vi "Configure_SL.vi"() -> (1 "changed?":bool, 2 "Property":string[](array[string]))   [LabVIEW 2019]
uses:
  <vilib>/Utility/miscctls.llb/LVRowAndColumnUnsignedTypeDef.ctl
panel:
  out "Table Control":string[][](table)
  out "error out":errorcluster
  in  "Properties":i32(listbox)=-1
  in  "Cancel":bool
  in  "OK":bool
  # "SystemLink Panel\n\nhttps://www.systemlinkcloud.com\n\nAPI: https://api.systemlinkcloud.com"
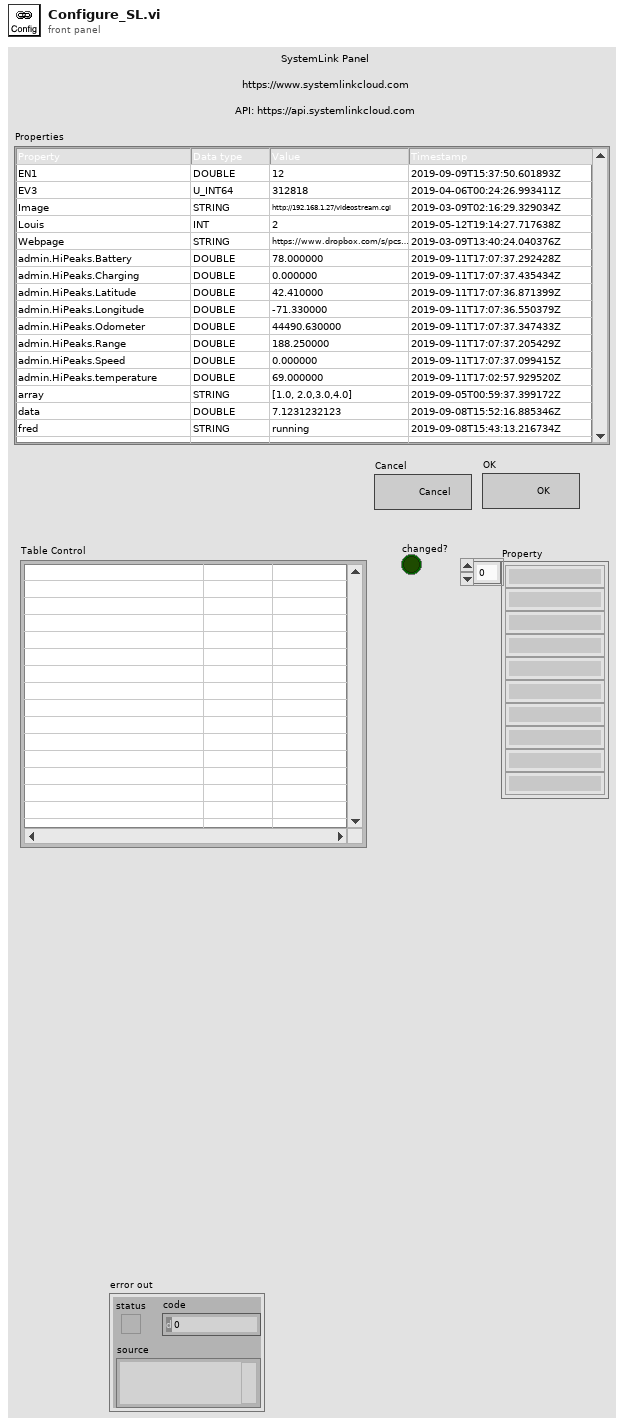
[diagram p1: front panel]
types:
  T1 = typedef "LVRowAndColumnUnsignedTypeDef.ctl" = cluster{"Row":u32, "Column":u32}
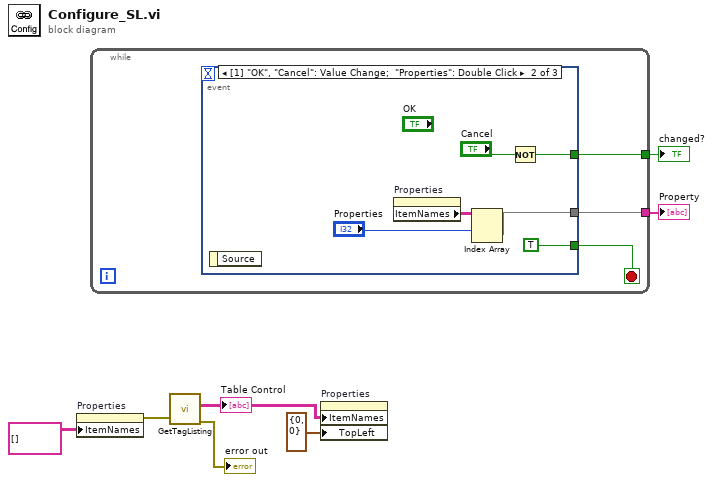
[diagram p0: block diagram]
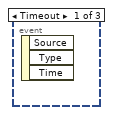
[diagram p2: hidden frame]
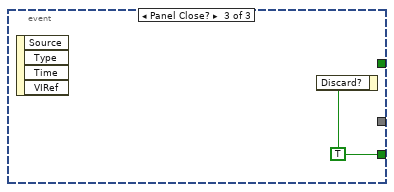
[diagram p3: hidden frame]
diagram:
  n1 = property on="Properties" class="MCListbox (strict)"("ItemNames"=string[][] [] ("Item Names")) -> (error out=w1:errorcluster)  [unwired: 2 in, 1 out]
  n2 = while {
    tunnel: [w10] -> w7
    tunnel: [w8] -> w6
    stop <- w9 stop-if-true
    n3 = event shown="[1] \"OK\", \"Cancel\": Value Change;  \"Properties\": Double Click" {
      selector: _ -> [_ _ _]
      dyn-events: _ -> [_ _ _]
      timeout: _ -> [_ _ _]
      tunnel: [_ w11 _] -> w10
      tunnel: [_ TRUE w17] -> w9
      tunnel: [_ w13 _] -> w8
      event Timeout {
        n4 = event-data() -> ()  [unwired: 1 in, 3 out]
      }
      event "OK", "Cancel": Value Change; "Properties": Double Click {
        n5 = event-data() -> ()  [unwired: 1 in, 1 out]
        n6 = property on="Properties" class="MCListbox (strict)"() -> ("ItemNames"=w15:string[][])  [unwired: 2 in, 2 out]
        n7 = Index Array(array=w15, index (row)="Properties") -> (element=w13:string[])  [unwired: 1 in]
        n8 = Not(x="Cancel") -> (.not. x?=w11:bool)
      }
      event Panel Close? {
        w17 = TRUE
        n9 = event-data() -> ()  [unwired: 1 in, 4 out]
        n10 = event-data("Discard?"=w17) -> ()  [unwired: 1 in, 1 out]
      }
    }
  }
  "changed?" <- w7
  "Property" <- w6
  n11 = call "GetTagListing.vi"("error in (no error)"=w1) -> ("error out"=→"error out":errorcluster, "info"=w4:string[][])  [unwired: 8 in, 1 out]
  "Table Control" <- w4
  n12 = property on="Properties" class="MCListbox (strict)"("ItemNames"=w4, "TopLeft"=T1 {"Row"=0, "Column"=0} ("Top Left Visible Cell")) -> ()  [unwired: 2 in, 2 out]
